vi "Example Extraction from JSON string.vi"() -> ()   [LabVIEW 2011]
doc: "Extracting data from JSON."
uses:
  vi.lib/Addons/JSON API/JSON Value/Set from JSON string.vi
  vi.lib/Addons/JSON API/JSON Value/Get as JSON string.vi
  vi.lib/Addons/JSON API/JSON Scalar/Get as Timestamp.vi
  vi.lib/Addons/JSON API/JSON Value/Get sub-Item by names.vi
  vi.lib/Addons/JSON API/JSON Array/Get Array.vi
  vi.lib/Addons/JSON API/JSON Value/Get Object Item by Name.vi
  vi.lib/Addons/JSON API/JSON Scalar/Get as DBL.vi
  vi.lib/Addons/JSON API/JSON Value/Get as JSON string (pretty).vi
  vi.lib/Addons/JSON API/JSON Value/Get Item by name array.vi
  vi.lib/Addons/JSON API/JSON Value/JSON Value.lvclass
  vi.lib/Addons/JSON API/Get Polymorphic/JSON GetSet.lvlib
  vi.lib/Addons/JSON API/JSON Scalar/JSON Scalar.lvclass
  vi.lib/Addons/JSON API/JSON Array/JSON Array.lvclass
panel:
  out "SubJSON":string
  out "T1 (alternate method)":dbl
  out "Alternate way of working with arrays":timestamp
  out "MixedArray as DBL (ignoring convertability errors)":dbl[](array[numeric])
  in  "JSON Input string":string="{\r  \"Nest\": {\r    \"MixedArray\": [\r      1.2,\r      \"Hi\",\r      \"2012-10-26T13:28:16.312Z\"\r    ],\r    \"DBLArray\": [\r      1.3,\r      2.4,\r      1.6\r    ],\r    \"ZZ\": 123\r  },\r  \"T1\": 456.789,\r  \"T2\": \"test2\"\r}"
  out "MixedArray extracted as JSON string":string
  out "T1":dbl
  out "element of mixed-type array":timestamp
  out "DBLArray from Nested Object":dbl[](array[numeric])
  # "see diagram"
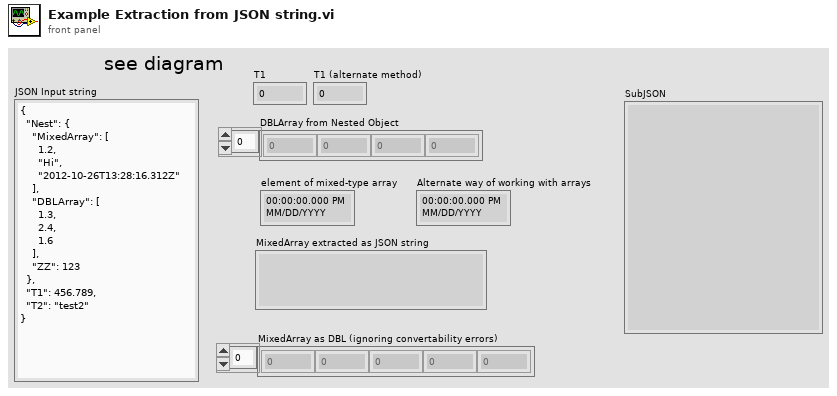
[diagram p1: front panel]
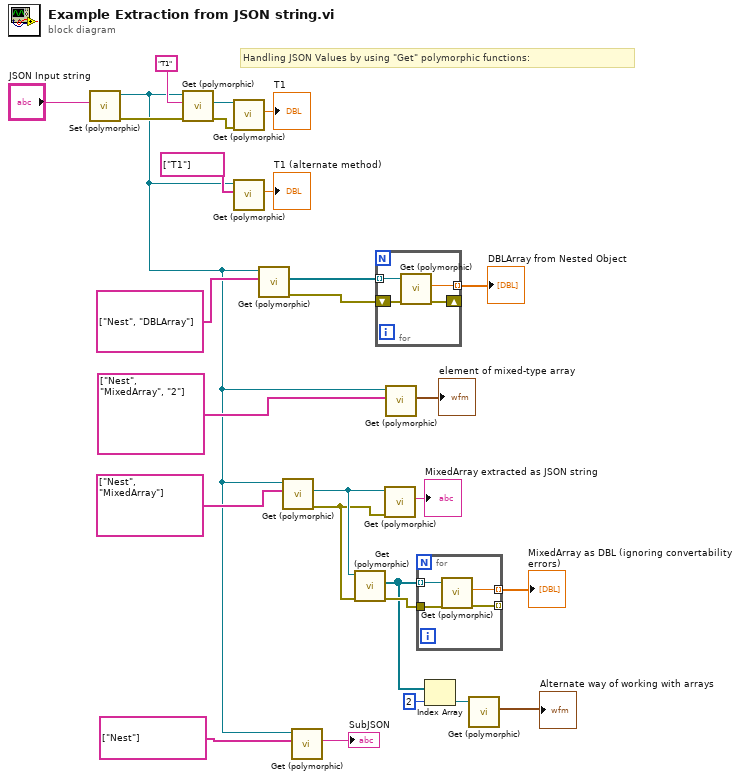
[diagram p0: block diagram]
diagram:
  # "Handling JSON Values by using \"Get\" polymorphic functions:"
  n1 = call-poly "Set (polymorphic).vi"("JSON stream"="JSON Input string") -> ("error out"=w27:errorcluster, "JSON Value out"=w3:refnum<class "JSON Value.lvclass">)  [unwired: 8 in, 1 out]
  n2 = call-poly "Get (polymorphic).vi"("error in (no error)"=w27, "name"="T1", "JSON Value In"=w3) -> ("error out"=w22:errorcluster, "Value"=w21:refnum<class "JSON Value.lvclass">)  [unwired: 5 in, 2 out]
  n3 = call-poly "Get (polymorphic).vi"("error in (no error)"=w22, "JSON Value in"=w21) -> ("Number"=→"T1":dbl)  [unwired: 7 in, 2 out]
  n4 = call-poly "Get (polymorphic).vi"("Name Array"=string[] ["T1"], "JSON Value in"=w3) -> ("Number"=→"T1 (alternate method)":dbl)  [unwired: 7 in, 2 out]
  n5 = call-poly "Get (polymorphic).vi"("Name Array"=string[] ["Nest", "DBLArray"], "JSON Array in"=w3) -> ("error out"=w7:errorcluster, "Array"=w8:refnum<class "JSON Value.lvclass">[])  [unwired: 7 in, 1 out]
  n6 = call-poly "Get (polymorphic).vi"("Name Array"=string[] ["Nest", "MixedArray"], "JSON Value In"=w3) -> ("error out"=w13:errorcluster, "Value"=w14:refnum<class "JSON Value.lvclass">)  [unwired: 6 in, 2 out]
  n7 = call-poly "Get (polymorphic).vi"("Name Array"=string[] ["Nest"], "JSON Value in"=w3) -> ("String"=→"SubJSON":string)  [unwired: 8 in, 1 out]
  n8 = call-poly "Get (polymorphic).vi"("error in (no error)"=w13, "JSON Array in"=w14) -> ("error out"=w16:errorcluster, "Array"=w12:refnum<class "JSON Value.lvclass">[])  [unwired: 7 in, 1 out]
  n9 = for {
    tunnel: w8 -> [w31] mode=indexing
    tunnel: [w30] -> w19 mode=indexing
    shift-right: [w28] -> _
    shift-left: w7 -> [w29]
    n10 = call-poly "Get (polymorphic).vi"("error in (no error)"=w29, "JSON Value in"=w31) -> ("error out"=w28:errorcluster, "Number"=w30:dbl)  [unwired: 7 in, 1 out]
  }
  "DBLArray from Nested Object" <- w19
  n11 = call-poly "Get (polymorphic).vi"("error in (no error)"=w13, "JSON Value in"=w14) -> ("String"=→"MixedArray extracted as JSON string":string)  [unwired: 8 in, 1 out]
  n12 = call-poly "Get (polymorphic).vi"("Name Array"=string[] ["Nest", "MixedArray", "2"], "JSON Value in"=w3) -> ("Time Stamp"=→"element of mixed-type array":timestamp)  [unwired: 7 in, 2 out]
  n13 = for {
    tunnel: w12 -> [w35] mode=indexing
    tunnel: [w34] -> w15 mode=indexing
    tunnel: w16 -> [w33]
    tunnel: [w32] -> _ mode=indexing
    n14 = call-poly "Get (polymorphic).vi"("error in (no error)"=w33, "JSON Value in"=w35) -> ("error out"=w32:errorcluster, "Number"=w34:dbl)  [unwired: 7 in, 1 out]
  }
  "MixedArray as DBL (ignoring convertability errors)" <- w15
  n15 = Index Array(array=w12, index=2) -> (element=w10:refnum<class "JSON Value.lvclass">)
  n16 = call-poly "Get (polymorphic).vi"("JSON Value in"=w10) -> ("Time Stamp"=→"Alternate way of working with arrays":timestamp)  [unwired: 8 in, 2 out]
